vi "Duplicate SBlock.vi"(8 "error in (no error)":errorcluster, 10 "index":i32, 11 "Sequence of SBlocks in":refnum<class "Sequence of SBlocks.lvclass">) -> (0 "error out":errorcluster, 3 "Sequence of SBlocks out":refnum<class "Sequence of SBlocks.lvclass">)   [LabVIEW 2020, in "Run Utilities.lvlib" / "Sequence of SBlocks.lvclass"]
uses:
  Sequence of SBlocks.lvclass
  Sequence of SBlocks.lvclass/Sequence of SBlocks.ctl
  Schedule Block/Schedule Block.lvclass
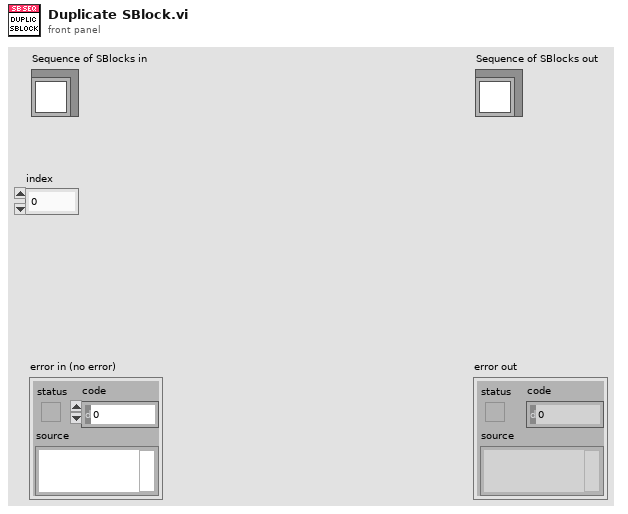
[diagram p1: front panel]
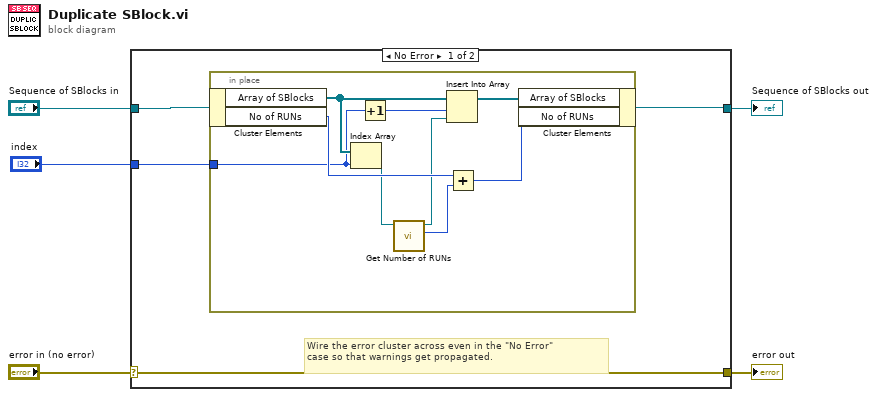
[diagram p0: block diagram]
diagram:
  n1 = case shown="No Error" "error in (no error)" {
    selector: "error in (no error)" -> [w9 w20]
    tunnel: [w9 w20] -> w4
    tunnel: [w7 w19] -> w2
    tunnel: "Sequence of SBlocks in" -> [w8 w19]
    tunnel: "index" -> [w6 _]
    frame No Error {
      # "Wire the error cluster across even in the \"No Error\"\ncase so that warnings get propagated."
      n2 = in-place {
        in-place-border: w6 -> [w11]
        n3 = in-place-cluster #1(w8) -> ("Array of SBlocks"=w14:refnum<class "Schedule Block.lvclass">[], "No of RUNs"=w16:i32)
        n4 = Index Array(array=w14, index=w11) -> (element=w13:refnum<class "Schedule Block.lvclass">)
        n5 = Increment(x=w11) -> (x+1=w10:i32)
        n6 = call-dynamic "Get Number of RUNs.vi"("Schedule Block in"=w13) -> ("No. of RUNs"=w17:i32, "Schedule Block out"=w12:refnum<class "Schedule Block.lvclass">)  [unwired: 8 in, 1 out]
        n7 = Insert Into Array(array=w14, index=w10, new element=w12) -> (w18:refnum<class "Schedule Block.lvclass">[])
        n8 = Add(x=w16, y=w17) -> (x+y=w15:i32)
        n9 = in-place-cluster #1("Array of SBlocks"=w18, "No of RUNs"=w15) -> (w7:refnum<class "Sequence of SBlocks.lvclass">)
      }
    }
    frame Error {
    }
  }
  "error out" <- w4
  "Sequence of SBlocks out" <- w2
